vi "Verify Cooler.vi"(8 "error in (no error)":errorcluster, 11 "Cooler in":refnum<class "Simulated_Cooler.lvclass">) -> (0 "error out":errorcluster, 2 "coolerStatus":bool, 3 "Cooler out":refnum<class "Simulated_Cooler.lvclass">)   [LabVIEW 2018, in "Simulated_Cooler.lvclass"]
uses:
  Simulated_Cooler.lvclass
  Simulated_Cooler.lvclass/Simulated_Cooler.ctl
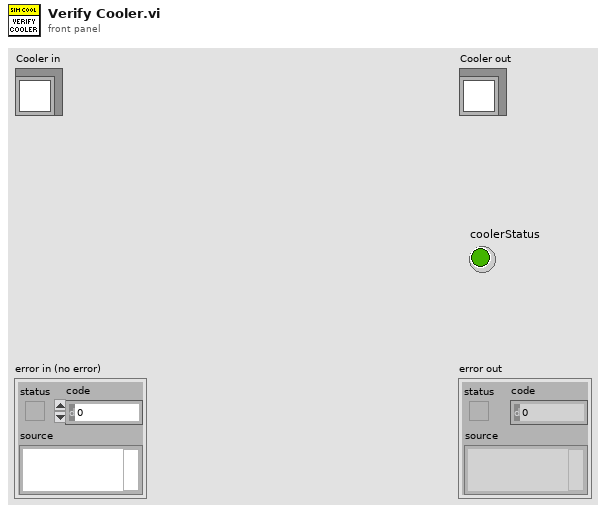
[diagram p1: front panel]
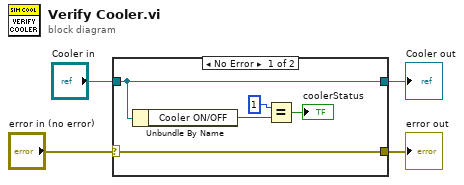
[diagram p0: block diagram]
diagram:
  n1 = case shown="No Error" "error in (no error)" {
    selector: "error in (no error)" -> [w9 w11]
    tunnel: [w9 w11] -> w1
    tunnel: [w6 w10] -> w3
    tunnel: "Cooler in" -> [w6 w10]
    frame No Error {
      n2 = Unbundle By Name(w6) -> ("Cooler ON/OFF"=w5:u8)
      n3 = Equal?(x=1, y=w5) -> (x = y?=→"coolerStatus":bool)
    }
    frame Error {
    }
  }
  "error out" <- w1
  "Cooler out" <- w3
